vi "Get Measurement Details.vi"(8 "error in":errorcluster, 11 "measurement plugin service in":refnum<class "Measurement Plugin Service.lvclass">) -> (0 "error out":errorcluster, 1 "service class":string, 2 "measurement details":T2, 3 "measurement plugin service out":refnum<class "Measurement Plugin Service.lvclass">, 4 "measurement annotations":T1[](array[typedef]))   [LabVIEW 2021, in "NI Measurement Plug-In SDK.lvlib" / "Measurement Plugin Service.lvclass"]
uses:
  Measurement Plugin Service.lvclass
  Helpers/TypeDefs/Measurement Details.ctl
  Helpers/TypeDefs/Measurement Annotation.ctl
  NI Measurement Plug-In SDK.lvlib
panel:
  # "This VI is marked as deprecated in favor of Get Service Descriptor.vi, retained solely for backward compatibility purposes."
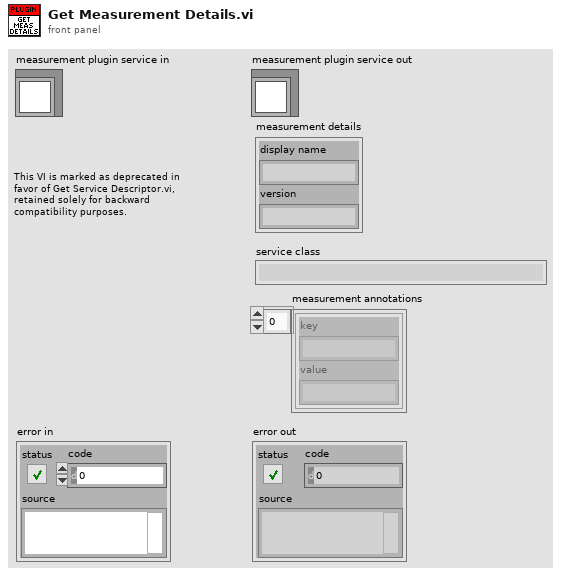
[diagram p1: front panel]
types:
  T1 = typedef "NI Measurement Plug-In SDK.lvlib/Measurement Annotation.ctl" = cluster{"key":string, "value":string}
  T2 = typedef "NI Measurement Plug-In SDK.lvlib/Measurement Details.ctl" = cluster{"display name":string, "version":string}
  T3 = typedef "NI Measurement Plug-In SDK.lvlib/Measurement Plugin Service.lvclass/Plugin Paths.ctl" = cluster{"get service descriptor VI path":path, "get type specializations VI path":path, "get UI details VI path":path, "measurement logic VI path":path, "measurement configuration ctl path":path, "measurement results ctl path":path}
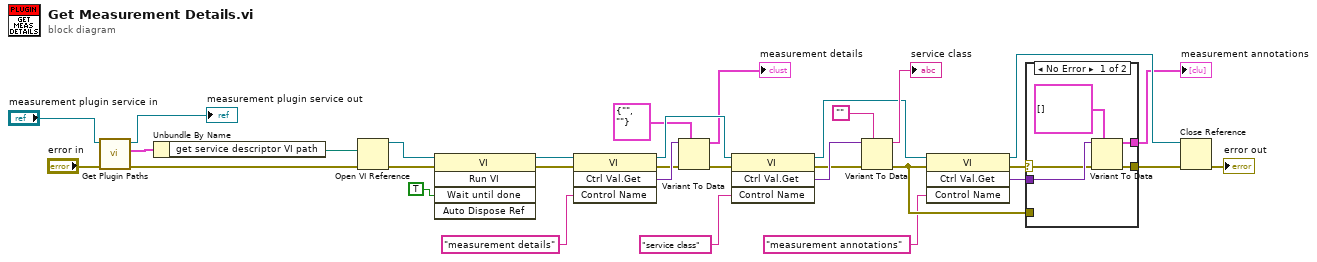
[diagram p0: block diagram]
diagram:
  n1 = call-dynamic "Get Plugin Paths.vi"("error in"="error in", "measurement plugin service in"="measurement plugin service in") -> ("error out"=w12:errorcluster, "plugin paths"=w29:T3, "measurement plugin service out"=→"measurement plugin service out":refnum<class "Measurement Plugin Service.lvclass">)  [unwired: 7 in]
  n2 = Unbundle By Name(w29) -> ("get service descriptor VI path"=w14:path)
  n3 = Open VI Reference(vi path=w14, error in (no error)=w12) -> (vi reference=w28:refnum<vi>, error out=w21:errorcluster)  [unwired: 4 in]
  n4 = invoke class="VI" method="Run VI"(reference=w28, error in=w21, "Wait until done"=TRUE ("Wait Until Done")) -> (reference out=w26:refnum<vi>, error out=w22:errorcluster)  [unwired: 2 in, 3 out]
  n5 = invoke class="VI" method="Ctrl Val.Get"(reference=w26, error in=w22, "Control Name"="measurement details") -> (reference out=w23:refnum<vi>, error out=w19:errorcluster, "Get Control Value Variant"=w20:variant)  [unwired: 1 in, 1 out]
  n6 = Variant To Data(error in=w19, type=T2 {"display name"="", "version"=""} ("MeasurementDetails"), Variant=w20) -> (data=→"measurement details":T2, error out=w18:errorcluster)
  n7 = invoke class="VI" method="Ctrl Val.Get"(reference=w23, error in=w18, "Control Name"="service class") -> (reference out=w7:refnum<vi>, error out=w16:errorcluster, "Get Control Value Variant"=w17:variant)  [unwired: 1 in, 1 out]
  n8 = Variant To Data(error in=w16, type="", Variant=w17) -> (data=→"service class":string, error out=w5:errorcluster)
  n9 = invoke class="VI" method="Ctrl Val.Get"(reference=w7, error in=w5, "Control Name"="measurement annotations") -> (reference out=w6:refnum<vi>, error out=w2:errorcluster, "Get Control Value Variant"=w4:variant)  [unwired: 1 in, 1 out]
  n10 = case shown="No Error" w2 {
    selector: w2 -> [w34 _]
    tunnel: [w37 w38] -> w8
    tunnel: w4 -> [w36 _]
    tunnel: [w35 _] -> w1
    tunnel: w5 -> [_ w38]
    frame No Error {
      n11 = Variant To Data(error in=w34, type=T1[] [], Variant=w36) -> (data=w35:T1[], error out=w37:errorcluster)
    }
    frame Error {
    }
  }
  "measurement annotations" <- w1
  n12 = Close Reference(reference=w6, error in (no error)=w8) -> (error out=→"error out":errorcluster)
